vi "Create I32ArrayMsg.vi"(8 "error in (no error)":errorcluster, 10 "Message Data":i32[](array[numeric]), 11 "Message Name":string) -> (0 "error out":errorcluster, 3 "I32ArrayMsg out":refnum<class "I32ArrayMsg.lvclass">)   [LabVIEW 2009, in "LapDog.Messaging.v2.NativeArrays.lvlib" / "I32ArrayMsg.lvclass"]
doc: "Returns an I32ArrayMsg object with the given name.\n\nThis method executes regardless of the error in state."
uses:
  I32ArrayMsg.lvclass
  I32ArrayMsg.lvclass/I32ArrayMsg.ctl
  Messaging.v2/MessageObject/Message.lvclass
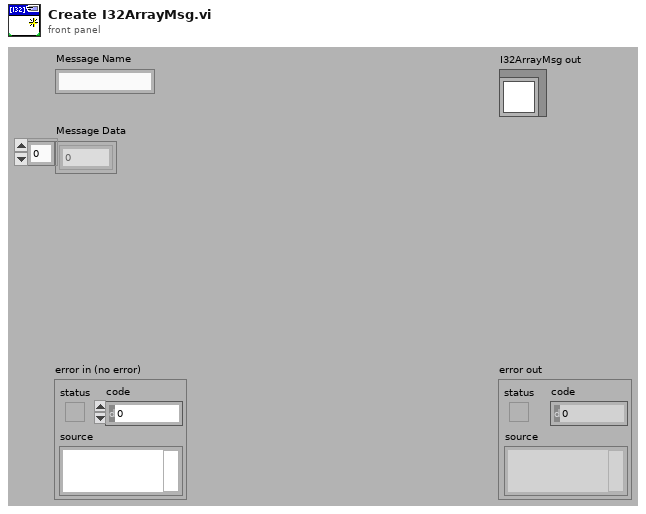
[diagram p1: front panel]
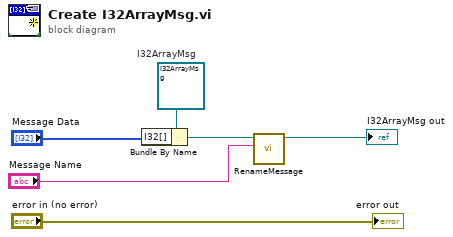
[diagram p0: block diagram]
diagram:
  w6 = refnum<class "I32ArrayMsg.lvclass"> refnum  # I32ArrayMsg
  n1 = Bundle By Name(cluster=w6, "I32[]"="Message Data") -> (w3:refnum<class "I32ArrayMsg.lvclass">)
  n2 = call "RenameMessage.vi"("Message Name"="Message Name", "Message in"=w3) -> ("Message out"=→"I32ArrayMsg out":refnum<class "I32ArrayMsg.lvclass">)  [unwired: 8 in, 1 out]
  "error out" <- "error in (no error)"
